vi "Get NetworkTime.vi"(8 "error in (no error)":errorcluster, 11 "NetworkImpairmentPluginBase in":refnum<class "NetworkImpairmentPluginBase.lvclass">) -> (0 "error out":errorcluster, 2 "dblNetImpTime":dbl[](array[numeric]), 3 "NetworkImpairmentPluginBase out":refnum<class "NetworkImpairmentPluginBase.lvclass">)   [LabVIEW 2017, in "NetworkImpairmentPlugins.lvlib" / "NetworkImpairmentPluginBase.lvclass"]
uses:
  NetworkImpairmentPluginBase.lvclass
  NetworkImpairmentPluginBase.lvclass/NetworkImpairmentPluginBase.ctl
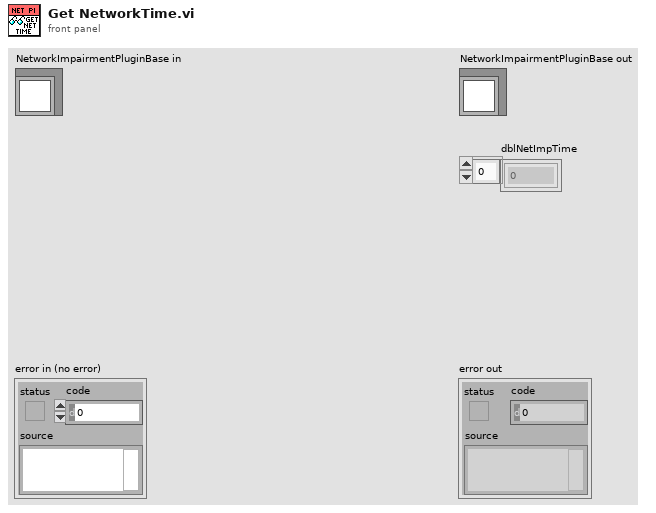
[diagram p1: front panel]
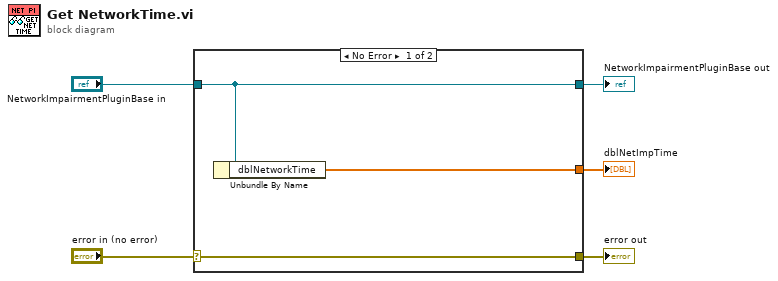
[diagram p0: block diagram]
diagram:
  n1 = case shown="No Error" "error in (no error)" {
    selector: "error in (no error)" -> [w8 w9]
    tunnel: [w8 w9] -> w4
    tunnel: [w7 w10] -> w2
    tunnel: "NetworkImpairmentPluginBase in" -> [w7 w10]
    tunnel: [w6 _] -> w1
    frame No Error {
      n2 = Unbundle By Name(w7) -> ("dblNetworkTime"=w6:dbl[])
    }
    frame Error {
    }
  }
  "error out" <- w4
  "NetworkImpairmentPluginBase out" <- w2
  "dblNetImpTime" <- w1
